vi "DDS Write RAM register 2.vi"(6 "channel number (1)":u8=1 min=1 max=4 step=1, 7 "Register":T3=enum."RAM", 8 "error in (no error)":errorcluster, 9 "# of Words":u16, 10 "Write Data":u8[][](array[numeric]), 11 "DDS ref in":T1={"NI USB-8451 device reference"="", "DIO port"=0, "Serial Clock Rate [kHz]"=1000}) -> (0 "error out":errorcluster, 3 "DDS ref out":T1={"NI USB-8451 device reference"="", "DIO port"=0, "Serial Clock Rate [kHz]"=1000})   [LabVIEW 2013]
uses:
  AD9910 registers.ctl
  DDS_box_device_reference.ctl
  <vilib>/ni845x/ni845x.llb/ni845xControl.ctl
panel:
  out "sent data":u8[][](array[numeric])
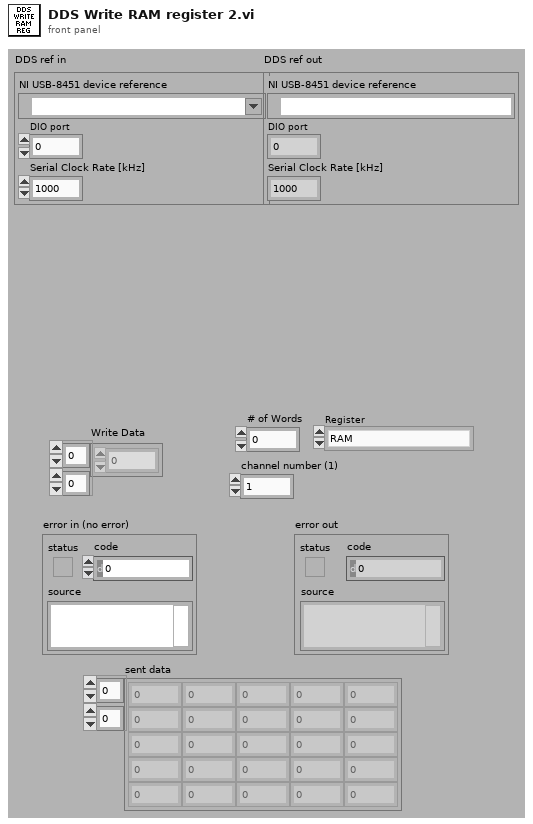
[diagram p1: front panel]
types:
  T1 = typedef "DDS_box_device_reference.ctl" = cluster{"NI USB-8451 device reference":T2, "DIO port":u8, "Serial Clock Rate [kHz]":u16}
  T2 = typedef "ni845xControl.ctl" = refnum<k21>
  T3 = typedef "AD9910 registers.ctl" = enum16{"CFR1", "CFR2", "CFR3", "Auxiliary DAC Control", "I/0 Update Rate", "Frequency Tuning Word", "Phase Offset Word", "Amplitude Scale Factor", "Multichip Sync", "Digital Ramp Limit", "Digital Ramp Step Size", "Digital Ramp Rate", "Single Tone Profile 0", "Single Tone Profile 1", "Single Tone Profile 2", "Single Tone Profile 3", "Single Tone Profile 4", "Single Tone Profile 5", "Single Tone Profile 6", "Single Tone Profile 7", "RAM Profile 0", "RAM Profile 1", "RAM Profile 2", "RAM Profile 3", "RAM Profile 4", "RAM Profile 5", "RAM Profile 6", "RAM Profile 7", "RAM"}
  T4 = typedef "ni845xSpiScriptControl.ctl" = refnum<k20>
  T5 = typedef "DDS CS pins.ctl" = enum8{"IO reset", "Ch. 4 CS", "Ch. 3 CS", "Ch. 2 CS", "Ch. 1 CS"}
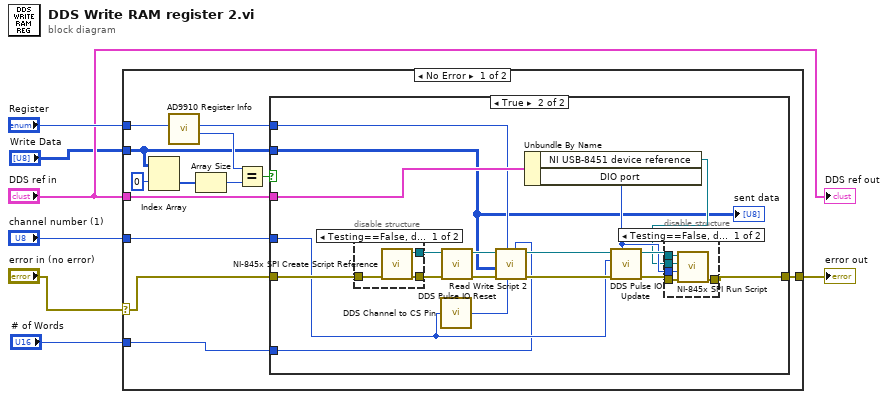
[diagram p0: block diagram]
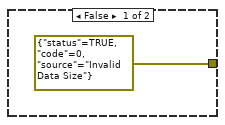
[diagram p2: hidden frame]
diagram:
  n1 = case shown="No Error" "error in (no error)" {
    selector: "error in (no error)" -> [w8 w50]
    tunnel: "DDS ref in" -> [w20 _]
    tunnel: "Register" -> [w19 _]
    tunnel: [w14 w50] -> w5
    tunnel: "Write Data" -> [w11 _]
    tunnel: "channel number (1)" -> [w13 _]
    tunnel: "# of Words" -> [w12 _]
    frame No Error {
      n2 = Index Array(array=w11, index (row)=0) -> (element=w9:u8[])  [unwired: 1 in]
      n3 = call "AD9910 Register Info.vi"("Register"=w19) -> ("Number of Bytes"=w18:i32, "Address"=w15:u8)  [unwired: 9 in]
      n4 = Array Size(array=w9) -> (size(s)=w17:i32)
      n5 = Equal?(x=w18, y=w17) -> (x = y?=w16:bool)
      n6 = case shown="True" w16 {
        tunnel: w8 -> [_ w39]
        tunnel: w20 -> [_ w38]
        tunnel: w11 -> [_ w22]
        tunnel: w15 -> [_ w24]
        tunnel: [errorcluster {"status"=TRUE, "code"=0, "source"="Invalid Data Size"} ("error in (no error)") w32] -> w14
        tunnel: w13 -> [_ w27]
        tunnel: w12 -> [_ w23]
        frame False {
        }
        frame True {
          n7 = disable-structure shown="Testing==False, default" {
            disable-tunnel: w39 -> [w48 w49]
            disable-tunnel: [w47 _] -> w37
            disable-tunnel: [w46 w49] -> w36
            frame condition #0 (active) {
              n8 = call <vilib>:"NI-845x SPI Create Script Reference.vi"("error in (no error)"=w48) -> ("error out"=w46:errorcluster, "spi script reference"=w47:T4)  [unwired: 9 in]
            }
            frame condition #1 {
            }
          }
          n9 = call "DDS Channel to CS Pin.vi"("channel number (1)"=w27) -> ("CS pin"=w28:T5)
          n10 = call "DDS Pulse IO Reset.vi"("error in (no error)"=w36, "spi script reference in"=w37) -> ("error out"=w33:errorcluster, "spi script reference out"=w34:T4)  [unwired: 8 in]
          n11 = call "Read Write Script 2.vi"("# of Words"=w23, "chip select (0)"=w28, "Write register"=w24, "error in (no error)"=w33, "Write Data"=w22, "spi script reference in"=w34) -> ("error out"=w31:errorcluster, "spi script reference out"=w35:T4)  [unwired: 3 in, 1 out]
          n12 = Unbundle By Name(w38) -> ("NI USB-8451 device reference"=w25:T2, "DIO port"=w26:u8)
          n13 = call "DDS Pulse IO Update.vi"("port number (0)"=w26, "error in (no error)"=w31, "channel number (1)"=w27, "spi script reference in"=w35) -> ("error out"=w30:errorcluster, "spi script reference out"=w29:T4)  [unwired: 6 in]
          n14 = disable-structure shown="Testing==False, default" {
            disable-tunnel: w25 -> [w44 _]
            disable-tunnel: [w43 w45] -> w32
            disable-tunnel: w29 -> [w42 _]
            disable-tunnel: w30 -> [w41 w45]
            disable-tunnel: w26 -> [w40 _]
            frame condition #0 (active) {
              n15 = call <vilib>:"NI-845x SPI Run Script.vi"("error in (no error)"=w41, "port (0)"=w40, "device reference in"=w44, "spi script reference in"=w42) -> ("error out"=w43:errorcluster)  [unwired: 5 in, 2 out]
            }
            frame condition #1 {
            }
          }
          "sent data" <- w22
        }
      }
    }
    frame Error {
    }
  }
  "error out" <- w5
  "DDS ref out" <- "DDS ref in"
